vi "Set Boolean.vi"(10 "Boolean Value":bool, 11 "Abs_Boolean.lvclass":refnum<class "Abs_Boolean.lvclass">) -> (3 "Node":refnum<class "bt_Node.lvclass">)   [LabVIEW 2021, in "BT AbsType.lvlib"]
uses:
  BT AbsType.lvlib
  Source/Support/Nodes/abs_Node/bt_Node.lvclass
  <vilib>/TSA/Abstract Data Classes/Abs_Types/Boolean/Abs_Boolean.lvclass
  C:/Program Files (x86)/National Instruments/LabVIEW 2021/vi.lib/TSA/Abstract Data Classes/Abs_Types/Type/Abs_Type.lvclass
  Set Boolean/Set Boolean.lvclass
  C:/Users/Tim/Documents/GitHub/LV_Behaviour_Tree/BT Abstract Type/abs_Type Leaf/abs_Type Leaf.lvclass
  C:/Users/Tim/Documents/GitHub/LV_Behaviour_Tree/Source/Support/Nodes/abs_Node/BT_Node.lvclass
  abs_Type Leaf/abs_Type Leaf.lvclass/abs_Type Leaf.ctl
  Set Boolean/Set Boolean.lvclass/Set Boolean.ctl
  abs_Type Leaf/Properties/Write Value Class.vi
  Set Boolean/Properties/Write Boolean.vi
  C:/Program Files (x86)/National Instruments/LabVIEW 2021/vi.lib/TSA/Abstract Data Classes/Abs_Types/Value/Abs_Value.lvclass
  C:/Program Files (x86)/National Instruments/LabVIEW 2021/vi.lib/TSA/Abstract Data Classes/Abs_Types/Boolean/Abs_Boolean.lvclass
  C:/Users/Tim/Documents/GitHub/LV_Behaviour_Tree/Source/Support/Nodes/Leaves/Leaf/bt_Leaf.lvclass
  C:/Users/Tim/Documents/GitHub/LV_Behaviour_Tree/Source/Support/Nodes/abs_Node/bt_Node.lvclass
  C:/Users/Tim/Documents/GitHub/LV_Behaviour_Tree/BT Abstract Type/Set Boolean/Set Boolean.lvclass
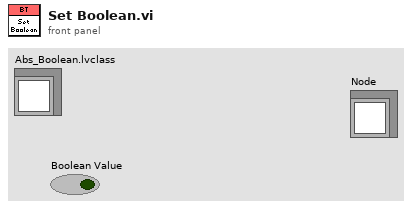
[diagram p1: front panel]
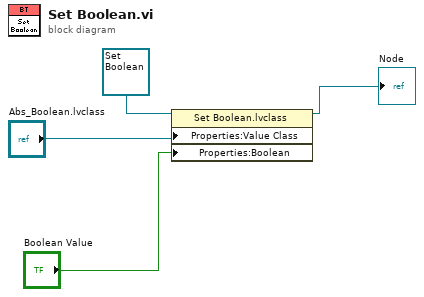
[diagram p0: block diagram]
diagram:
  n1 = property class="Set Boolean.lvclass"(reference=refnum<class "Set Boolean.lvclass"> refnum ("BT.lvlib:Set Boolean.lvclass"), "Properties:Value Class"="Abs_Boolean.lvclass", "Properties:Boolean"="Boolean Value") -> (reference out=→"Node":refnum<class "Set Boolean.lvclass">)  [unwired: 1 in, 1 out]
